vi "GDSString_ChangeToBetterNames.vi"(10 "NameIn":string) -> (1 "Changed":bool, 2 "NameOut":string)   [LabVIEW 2016]
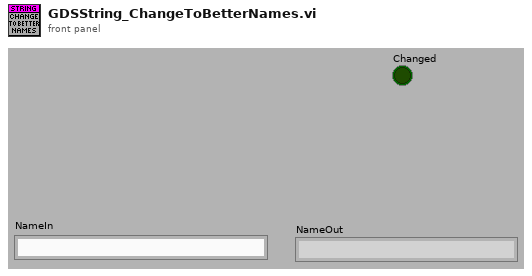
[diagram p1: front panel]
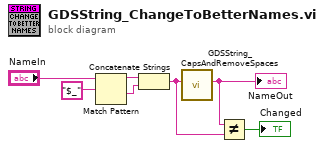
[diagram p0: block diagram]
diagram:
  n1 = Match Pattern(string="NameIn", regular expression="$_") -> (before substring=w4:string, after substring=w7:string)  [unwired: 1 in, 2 out]
  n2 = Concatenate Strings(w4, w7) -> (w2:string)
  n3 = call <resource>:"GDSString_CapsAndRemoveSpaces.vi"("String"=w2) -> ("concatenated string"=w3:string)  [unwired: 10 in]
  "NameOut" <- w3
  n4 = Not Equal?(x=w3, y=w2) -> (x != y?=→"Changed":bool)
